vi "setSuperKControlEmission.vi"(6 "error in (no error)":errorcluster, 8 "emission":u8, 9 "COMport":string="COM6") -> (0 "error out":errorcluster)   [LabVIEW 2015]
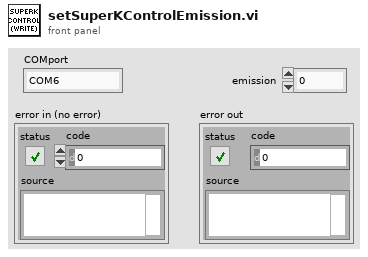
[diagram p1: front panel]
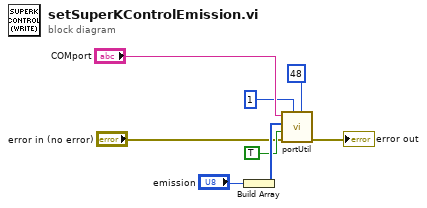
[diagram p0: block diagram]
diagram:
  n1 = Build Array("emission") -> (w7:u8[])
  n2 = call "portUtil.vi"("Register"=u8 48, "Destination"=u8 1, "error in (no error)"="error in (no error)", "WriteNotRead"=TRUE, "Array"=w7, "COMport"="COMport") -> ("error out"=→"error out":errorcluster)  [unwired: 3 in, 2 out]
